vi "Plate Configuration_new.vi"(7 "all rows":string[][](array[string])=[["", "Well", "Fluor", "Target", "Content", "Sample", "Cq", "SQ"], ["", "A01", "SYBR", "Fos", "Unkn", "Fl1", "23.40", ""], ["", "A02", "SYBR", "Fos", "Unkn", "Fl1", "23.24", ""], ["", "A03", "SYBR", "Fos", "Unkn", "Fl2", "23.55", ""], ["", "A04", "SYBR", "Fos", "Unkn", "Fl2", "23.53", ""], ["", "A05", "SYBR", "Fos", "Unkn", "Fl3", "23.38", ""], ["", "A06", "SYBR", "Fos", "Unkn", "Fl3", "23.50", ""], ["", "A07", "SYBR", "Fos", "Unkn", "Pfl1", "22.43", ""], ["", "A08", "SYBR", "Fos", "Unkn", "Pfl1", "22.94", ""], ["", "A09", "SYBR", "Fos", "Unkn", "Pfl2", "21.10", ""], ["", "A10", "SYBR", "Fos", "Unkn", "Pfl2", "21.46", ""], ["", "A11", "SYBR", "Fos", "Unkn", "Pfl3", "22.49", ""], ["", "A12", "SYBR", "Fos", "Unkn", "Pfl3", "22.89", ""], ["", "B01", "SYBR", "Arc", "Unkn", "Fl1", "32.28", ""], ["", "B02", "SYBR", "Arc", "Unkn", "Fl1", "32.59", ""], ["", "B03", "SYBR", "Arc", "Unkn", "Fl2", "32.93", ""], ["", "B04", "SYBR", "Arc", "Unkn", "Fl2", "32.78", ""], ["", "B05", "SYBR", "Arc", "Unkn", "Fl3", "32.38", ""], ["", "B06", "SYBR", "Arc", "Unkn", "Fl3", "32.35", ""], ["", "B07", "SYBR", "Arc", "Unkn", "Pfl1", "30.44", ""], ["", "B08", "SYBR", "Arc", "Unkn", "Pfl1", "30.58", ""], ["", "B09", "SYBR", "Arc", "Unkn", "Pfl2", "30.07", ""], ["", "B10", "SYBR", "Arc", "Unkn", "Pfl2", "30.20", ""], ["", "B11", "SYBR", "Arc", "Unkn", "Pfl3", "30.38", ""], ["", "B12", "SYBR", "Arc", "Unkn", "Pfl3", "30.04", ""], ["", "C01", "SYBR", "Jun", "Unkn", "Fl1", "25.27", ""], ["", "C02", "SYBR", "Jun", "Unkn", "Fl1", "24.72", ""], ["", "C03", "SYBR", "Jun", "Unkn", "Fl2", "25.47", ""], ["", "C04", "SYBR", "Jun", "Unkn", "Fl2", "25.79", ""], ["", "C05", "SYBR", "Jun", "Unkn", "Fl3", "25.27", ""], ["", "C06", "SYBR", "Jun", "Unkn", "Fl3", "25.52", ""], ["", "C07", "SYBR", "Jun", "Unkn", "Pfl1", "23.53", ""], ["", "C08", "SYBR", "Jun", "Unkn", "Pfl1", "23.37", ""], ["", "C09", "SYBR", "Jun", "Unkn", "Pfl2", "21.29", ""], ["", "C10", "SYBR", "Jun", "Unkn", "Pfl2", "38.35", ""], ["", "C11", "SYBR", "Jun", "Unkn", "Pfl3", "23.20", ""], ["", "C12", "SYBR", "Jun", "Unkn", "Pfl3", "23.23", ""], ["", "D01", "SYBR", "JunB", "Unkn", "Fl1", "26.08", ""], ["", "D02", "SYBR", "JunB", "Unkn", "Fl1", "26.09", ""], ["", "D03", "SYBR", "JunB", "Unkn", "Fl2", "27.02", ""], ["", "D04", "SYBR", "JunB", "Unkn", "Fl2", "27.08", ""], ["", "D05", "SYBR", "JunB", "Unkn", "Fl3", "26.91", ""], ["", "D06", "SYBR", "JunB", "Unkn", "Fl3", "26.93", ""], ["", "D07", "SYBR", "JunB", "Unkn", "Pfl1", "25.32", ""], ["", "D08", "SYBR", "JunB", "Unkn", "Pfl1", "25.12", ""], ["", "D09", "SYBR", "JunB", "Unkn", "Pfl2", "24.28", ""], ["", "D10", "SYBR", "JunB", "Unkn", "Pfl2", "24.21", ""], ["", "D11", "SYBR", "JunB", "Unkn", "Pfl3", "25.01", ""], ["", "D12", "SYBR", "JunB", "Unkn", "Pfl3", "25.38", ""], ["", "E01", "SYBR", "Ctgf", "Unkn", "Fl1", "27.57", ""], ["", "E02", "SYBR", "Ctgf", "Unkn", "Fl1", "27.52", ""], ["", "E03", "SYBR", "Ctgf", "Unkn", "Fl2", "28.24", ""], ["", "E04", "SYBR", "Ctgf", "Unkn", "Fl2", "28.02", ""], ["", "E05", "SYBR", "Ctgf", "Unkn", "Fl3", "28.10", ""], ["", "E06", "SYBR", "Ctgf", "Unkn", "Fl3", "27.90", ""], ["", "E07", "SYBR", "Ctgf", "Unkn", "Pfl1", "25.17", ""], ["", "E08", "SYBR", "Ctgf", "Unkn", "Pfl1", "25.51", ""], ["", "E09", "SYBR", "Ctgf", "Unkn", "Pfl2", "25.49", ""], ["", "E10", "SYBR", "Ctgf", "Unkn", "Pfl2", "25.43", ""], ["", "E11", "SYBR", "Ctgf", "Unkn", "Pfl3", "25.45", ""], ["", "E12", "SYBR", "Ctgf", "Unkn", "Pfl3", "25.45", ""], ["", "F01", "SYBR", "Nr4a1", "Unkn", "Fl1", "25.09", ""], ["", "F02", "SYBR", "Nr4a1", "Unkn", "Fl1", "25.24", ""], ["", "F03", "SYBR", "Nr4a1", "Unkn", "Fl2", "26.15", ""], ["", "F04", "SYBR", "Nr4a1", "Unkn", "Fl2", "26.01", ""], ["", "F05", "SYBR", "Nr4a1", "Unkn", "Fl3", "26.17", ""], ["", "F06", "SYBR", "Nr4a1", "Unkn", "Fl3", "26.29", ""], ["", "F07", "SYBR", "Nr4a1", "Unkn", "Pfl1", "24.23", ""], ["", "F08", "SYBR", "Nr4a1", "Unkn", "Pfl1", "24.26", ""], ["", "F09", "SYBR", "Nr4a1", "Unkn", "Pfl2", "23.05", ""], ["", "F10", "SYBR", "Nr4a1", "Unkn", "Pfl2", "23.08", ""], ["", "F11", "SYBR", "Nr4a1", "Unkn", "Pfl3", "24.02", ""], ["", "F12", "SYBR", "Nr4a1", "Unkn", "Pfl3", "24.04", ""], ["", "G01", "SYBR", "Egr1", "Unkn", "Fl1", "26.85", ""], ["", "G02", "SYBR", "Egr1", "Unkn", "Fl1", "26.59", ""], ["", "G03", "SYBR", "Egr1", "Unkn", "Fl2", "27.75", ""], ["", "G04", "SYBR", "Egr1", "Unkn", "Fl2", "27.76", ""], ["", "G05", "SYBR", "Egr1", "Unkn", "Fl3", "27.92", ""], ["", "G06", "SYBR", "Egr1", "Unkn", "Fl3", "28.27", ""], ["", "G07", "SYBR", "Egr1", "Unkn", "Pfl1", "25.19", ""], ["", "G08", "SYBR", "Egr1", "Unkn", "Pfl1", "24.90", ""], ["", "G09", "SYBR", "Egr1", "Unkn", "Pfl2", "23.36", ""], ["", "G10", "SYBR", "Egr1", "Unkn", "Pfl2", "23.81", ""], ["", "G11", "SYBR", "Egr1", "Unkn", "Pfl3", "24.67", ""], ["", "G12", "SYBR", "Egr1", "Unkn", "Pfl3", "24.81", ""], ["", "H01", "SYBR", "beta-Actin", "Unkn", "Fl1", "22.22", ""], ["", "H02", "SYBR", "beta-Actin", "Unkn", "Fl1", "22.27", ""], ["", "H03", "SYBR", "beta-Actin", "Unkn", "Fl2", "22.94", ""], ["", "H04", "SYBR", "beta-Actin", "Unkn", "Fl2", "22.82", ""], ["", "H05", "SYBR", "beta-Actin", "Unkn", "Fl3", "23.04", ""], ["", "H06", "SYBR", "beta-Actin", "Unkn", "Fl3", "22.72", ""], ["", "H07", "SYBR", "beta-Actin", "Unkn", "Pfl1", "22.09", ""], ["", "H08", "SYBR", "beta-Actin", "Unkn", "Pfl1", "22.09", ""], ["", "H09", "SYBR", "beta-Actin", "Unkn", "Pfl2", "21.57", ""], ["", "H10", "SYBR", "beta-Actin", "Unkn", "Pfl2", "21.16", ""], ["", "H11", "SYBR", "beta-Actin", "Unkn", "Pfl3", "21.80", ""], ["", "H12", "SYBR", "beta-Actin", "Unkn", "Pfl3", "21.93", ""]] caption="모든 행") -> (0 "출력 클러스터":T4, 1 "RowHdrs":string[](array[string]), 2 "Internal Ctrl":string[][](array[string]), 3 "Target Gene":string[][][](array[string]))   [LabVIEW 2015]
uses:
  <vilib>/Utility/config.llb/NI_LVConfig.lvlib
panel:
  in  "12":string="KO3"
  in  "11":string="KO3"
  in  "10":string="WT3"
  in  "09":string="WT3"
  in  "08":string="KO2"
  in  "07":string="KO2"
  in  "06":string="WT2"
  in  "05":string="WT2"
  in  "04":string="KO1"
  in  "03":string="KO1"
  in  "02":string="WT1"
  in  "01":string="WT1"
  in  "ColLabel":T1(array[ring])=[enum."11", enum."11", enum."21", enum."21", enum."12", enum."12", enum."22", enum."22", enum."13", enum."13", enum."23", enum."23"]
  out "RowLabel":T2(array[cluster])
  in  "H":string="H"
  in  "G":string="G"
  in  "F":string="F"
  in  "E":string="E"
  in  "D":string="D"
  in  "C":string="C"
  in  "B":string="B"
  in  "RowLabel":T3(array[ring])
  in  "A":string="A"
  in  "출력 클러스터 2":T4={"Group #"=2.0, "Biological replicate"=3.0, "Technical replicate"=2.0}
  out "ColLabel (C)":T5(array[cluster])=[{"ColNames"="01", "Label"=enum."11"}, {"ColNames"="02", "Label"=enum."11"}, {"ColNames"="03", "Label"=enum."12"}, {"ColNames"="04", "Label"=enum."12"}, {"ColNames"="05", "Label"=enum."13"}, {"ColNames"="06", "Label"=enum."13"}, {"ColNames"="07", "Label"=enum."21"}, {"ColNames"="08", "Label"=enum."21"}, {"ColNames"="09", "Label"=enum."22"}, {"ColNames"="10", "Label"=enum."22"}, {"ColNames"="11", "Label"=enum."23"}, {"ColNames"="12", "Label"=enum."23"}]
  in  "정지":bool
  # "Sample"
  # "Label"
  # "Gene Name"
  # "Label"
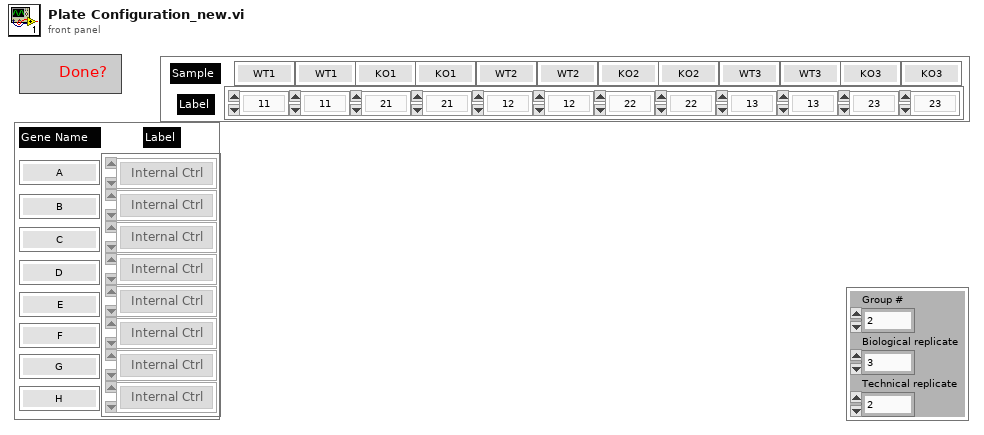
[diagram p1: front panel]
types:
  T1 = enum16{"11", "12", "13", "21", "22", "23", "Empty"}[]
  T2 = cluster{"H":string, "Label":enum16{"Empty Ch", "Target Ch", "Internal Ctrl"}}[]
  T3 = enum16{"Empty Ch", "Target Ch", "Internal Ctrl"}[]
  T4 = cluster{"Group #":dbl, "Biological replicate":dbl, "Technical replicate":dbl}
  T5 = cluster{"ColNames":string, "Label":enum16{"11", "12", "13", "21", "22", "23", "Empty"}}[]
  T6 = typedef "NI_LVConfig.lvlib/Config Data RefNum.ctl" = refnum<k1>
  T7 = cluster{"H":string, "Label":enum16{"Empty Ch", "Target Ch", "Internal Ctrl"}}
  T8 = cluster{"12":string, "Label":enum16{"11", "12", "13", "21", "22", "23", "Empty"}}
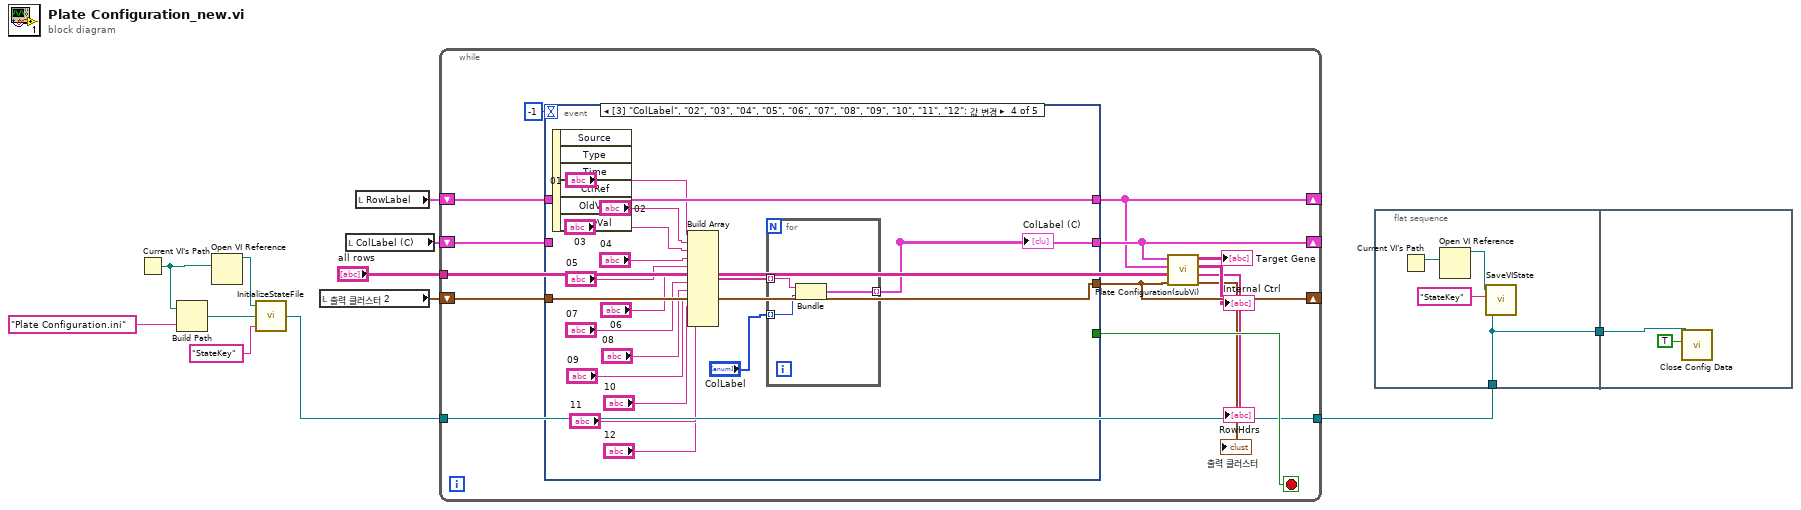
[diagram p0: block diagram]
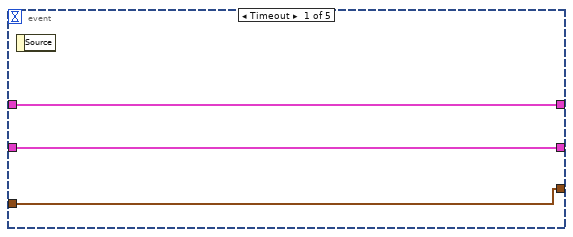
[diagram p2: hidden frame]
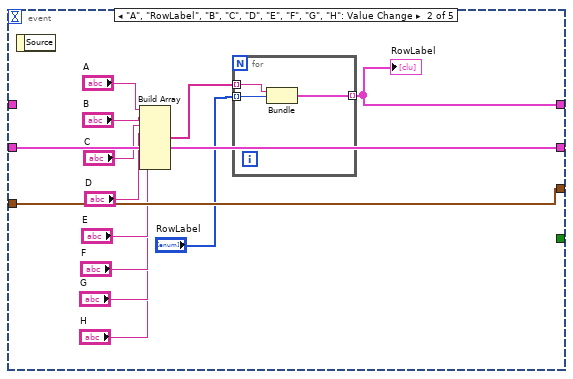
[diagram p3: hidden frame]
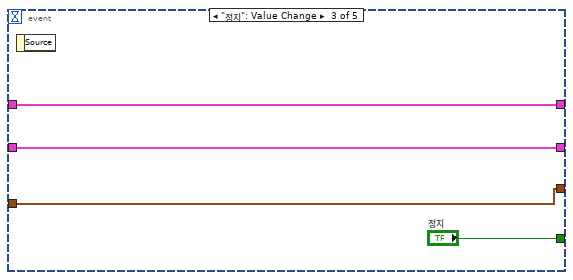
[diagram p4: hidden frame]
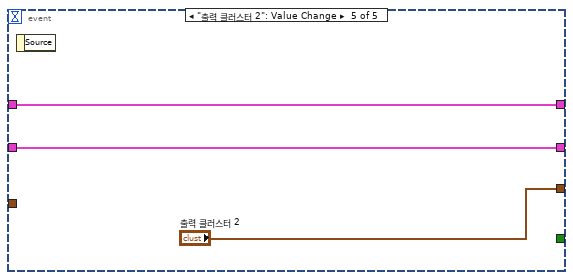
[diagram p5: hidden frame]
diagram:
  n1 = Current VI's Path ("Current VI Path...")() -> (path=w4:path)
  n2 = Build Path(base path=w4, name or relative path="Plate Configuration.ini") -> (appended path=w5:path)
  n3 = Open VI Reference(vi path=w4) -> (vi reference=w7:refnum<vi>)  [unwired: 5 in, 1 out]
  n4 = call "InitializeStateFile.vi"("key"="StateKey", "configuration file path"=w5, "VI Refnum"=w7) -> ("StateFileRefnum"=w3:T6)
  n5 = local read "출력 클러스터 2"() -> (w10:T4)
  n6 = local read "ColLabel (C)"() -> (w11:T5)
  n7 = local read "RowLabel"() -> (w9:T2)
  n8 = while {
    shift-right: [w21] -> _
    shift-left: w9 -> [w25]
    shift-right: [w22] -> _
    shift-left: w11 -> [w24]
    shift-right: [w20] -> _
    shift-left: w10 -> [w19]
    tunnel: "all rows" -> [w14]
    tunnel: w3 -> [w13]
    tunnel: [w13] -> w2
    stop <- w23 stop-if-true
    n9 = event shown="[3] \"ColLabel\", \"02\", \"03\", \"04\", \"05\", \"06\", \"07\", \"08\", \"09\", \"10\", \"11\", \"12\": 값 변경" {
      selector: _ -> [_ _ _ _ _]
      dyn-events: _ -> [_ _ _ _ _]
      timeout: -1 -> [_ _ _ _ _]
      tunnel: [w29 w30 w48 w66 w72] -> w21
      tunnel: [w28 w42 w47 w50 w71] -> w22
      tunnel: w25 -> [w29 _ w48 w66 w72]
      tunnel: w24 -> [w28 w42 w47 _ w71]
      tunnel: [_ _ "정지" _ _] -> w23
      tunnel: [w27 w41 w46 w65 "출력 클러스터 2"] -> w20
      tunnel: w19 -> [w27 w41 w46 w65 _]
      event Timeout {
        n10 = event-data() -> ()  [unwired: 1 in, 1 out]
      }
      event "A", "RowLabel", "B", "C", "D", "E", "F", "G", "H": Value Change {
        n11 = event-data() -> ()  [unwired: 1 in, 1 out]
        n12 = Build Array("A", "B", "C", "D", "E", "F", "G", "H") -> (w32:string[])
        n13 = for {
          tunnel: w32 -> [w45] mode=indexing
          tunnel: "RowLabel" -> [w44] mode=indexing
          tunnel: [w43] -> w30 mode=indexing
          n14 = Bundle("H"=w45, "Label"=w44) -> (w43:T7)  [unwired: 1 in]
        }
        "RowLabel" <- w30
      }
      event "정지": Value Change {
        n15 = event-data() -> ()  [unwired: 1 in, 1 out]
      }
      event "ColLabel", "02", "03", "04", "05", "06", "07", "08", "09", "10", "11", "12": Value Change {
        n16 = event-data() -> ()  [unwired: 1 in, 6 out]
        n17 = Build Array("01", "02", "03", "04", "05", "06", "07", "08", "09", "10", "11", "12") -> (w51:string[])
        n18 = for {
          tunnel: "ColLabel" -> [w68] mode=indexing
          tunnel: w51 -> [w69] mode=indexing
          tunnel: [w67] -> w50 mode=indexing
          n19 = Bundle("12"=w69, "Label"=w68) -> (w67:T8)  [unwired: 1 in]
        }
        "ColLabel (C)" <- w50
      }
      event "출력 클러스터 2": Value Change {
        n20 = event-data() -> ()  [unwired: 1 in, 1 out]
      }
    }
    n21 = call "Plate Configuration(subVi).vi"("출력 클러스터 2"=w20, "all rows"=w14, "RowLabel"=w21, "ColLabel"=w22) -> ("출력 클러스터"=→"출력 클러스터":T4, "RowHdrs"=→"RowHdrs":string[], "Internal Ctrl"=→"Internal Ctrl":string[][], "Target Gene"=→"Target Gene":string[][][])
  }
  n22 = flat-sequence {
    tunnel: w2 -> [w73]
    tunnel: [w73] -> w1
    tunnel: w1 -> [w77]
    frame #0 {
      n23 = Current VI's Path ("Current VI's Path...")() -> (path=w76:path)
      n24 = Open VI Reference(vi path=w76) -> (vi reference=w75:refnum<vi>)  [unwired: 5 in, 1 out]
      n25 = call "SaveVIState.vi"("StateFileRefnum"=w73, "key"="StateKey", "VI Refnum"=w75) -> ()
    }
    frame #1 {
      n26 = call <vilib>:"Close Config Data.vi"("write file if changed (T)"=TRUE ("write configuration file? (F)"), "refnum"=w77) -> ()  [unwired: 8 in, 2 out]
    }
  }
